vi "method1.vi"(8 "error in (no error)":errorcluster, 11 "ContentClass in":refnum<class "ContentClass.lvclass">) -> (0 "error out":errorcluster, 2 "RefNum":i32, 3 "ContentClass out":refnum<class "ContentClass.lvclass">)   [LabVIEW 2019, in "lv-providershell-example3.lvlib" / "ContentClass.lvclass"]
uses:
  ContentClass.lvclass
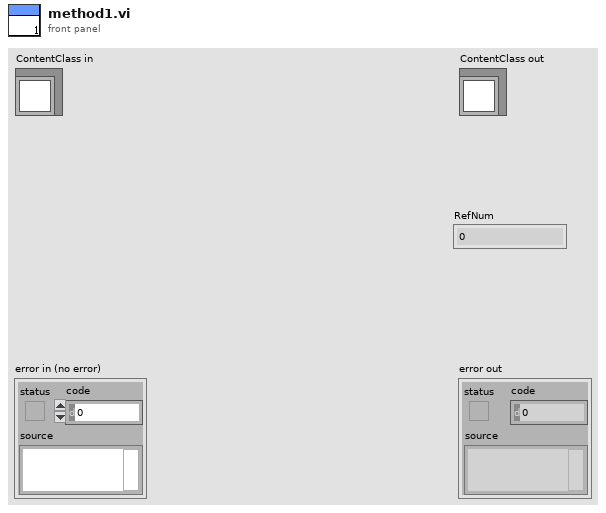
[diagram p1: front panel]
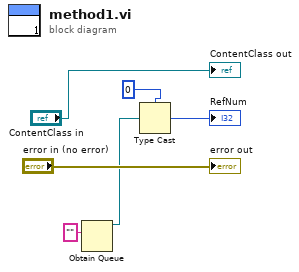
[diagram p0: block diagram]
diagram:
  n1 = Obtain Queue(element data type="" ("name (unnamed)")) -> (queue out=w3:refnum<queue>)  [unwired: 4 in, 2 out]
  n2 = Type Cast(type=0 ("RefNum"), x=w3) -> (*(type *) &x=→"RefNum":i32)
  "error out" <- "error in (no error)"
  "ContentClass out" <- "ContentClass in"
